vi "HGF_DIMService.appendData2Variant.vi"(0 "initData":variant, 1 "typeDescriptor":string, 2 "defaultData":string, 3 "defaultQuality":i32, 5 "error in (no error)":errorcluster) -> (14 "dup initData":variant, 19 "error out":errorcluster)   [LabVIEW 2012, in "HGF_DIM.lvlib" / "HGF_DIMService.lvclass"]
uses:
  HGF_DIMService.lvclass
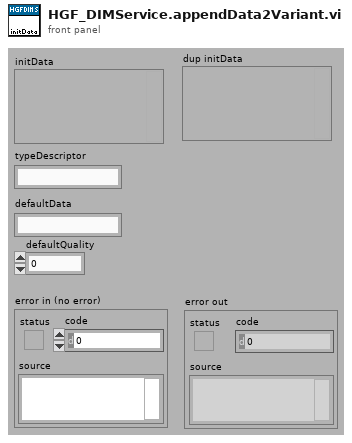
[diagram p1: front panel]
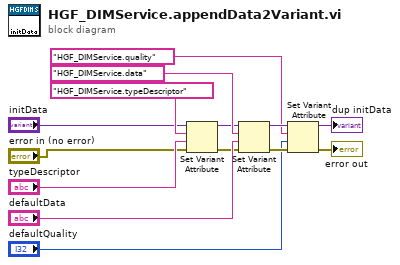
[diagram p0: block diagram]
diagram:
  n1 = Set Variant Attribute(Variant="initData", name="HGF_DIMService.typeDescriptor", value="typeDescriptor", error in="error in (no error)") -> (Variant out=w6:variant, error out=w5:errorcluster)  [unwired: 1 out]
  n2 = Set Variant Attribute(Variant=w6, name="HGF_DIMService.data", value="defaultData", error in=w5) -> (Variant out=w11:variant, error out=w12:errorcluster)  [unwired: 1 out]
  n3 = Set Variant Attribute(Variant=w11, name="HGF_DIMService.quality", value="defaultQuality", error in=w12) -> (Variant out=→"dup initData":variant, error out=→"error out":errorcluster)  [unwired: 1 out]
